vi "Set Grid Value Using Coordinates.vi"(6 "Cell Value":bool, 8 "error in (no error)":errorcluster, 9 "Row":u32, 10 "Column":u32, 11 "Grid Screen in":refnum<class "Grid Screen.lvclass">) -> (0 "error out":errorcluster, 3 "Grid Screen out":refnum<class "Grid Screen.lvclass">)   [LabVIEW 2024, in "Grid Screen.lvlib" / "Grid Screen.lvclass"]
uses:
  Grid Screen.lvclass
  Grid Screen.lvclass/Grid Screen.ctl
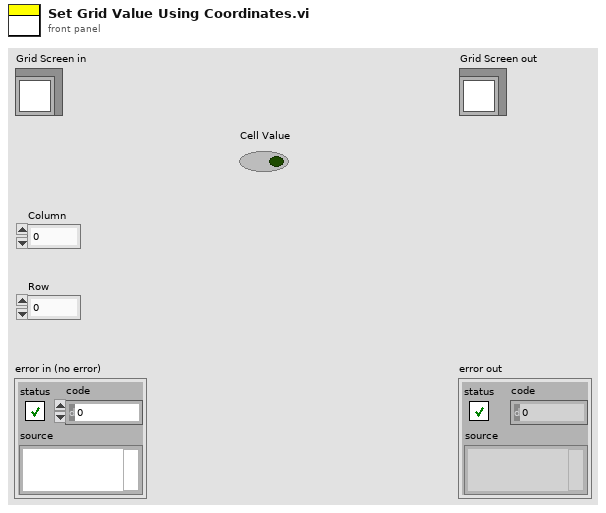
[diagram p1: front panel]
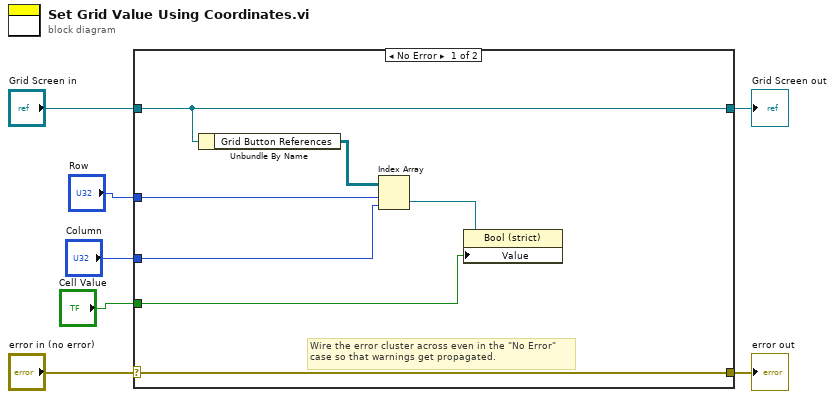
[diagram p0: block diagram]
diagram:
  n1 = case shown="No Error" "error in (no error)" {
    selector: "error in (no error)" -> [w14 w16]
    tunnel: [w14 w16] -> w6
    tunnel: [w13 w15] -> w4
    tunnel: "Grid Screen in" -> [w13 w15]
    tunnel: "Row" -> [w11 _]
    tunnel: "Column" -> [w10 _]
    tunnel: "Cell Value" -> [w8 _]
    frame No Error {
      # "Wire the error cluster across even in the \"No Error\"\ncase so that warnings get propagated."
      n2 = Unbundle By Name(w13) -> ("Grid Button References"=w12:refnum<vi>[][])
      n3 = Index Array(array=w12, index (row)=w11, index (col)=w10) -> (element=w9:refnum<vi>)
      n4 = property class="Bool (strict)"(reference=w9, "Value"=w8) -> ()  [unwired: 1 in, 2 out]
    }
    frame Error {
    }
  }
  "error out" <- w6
  "Grid Screen out" <- w4
